vi "Default Instrument Setup.vi"(8 "error in (no error)":errorcluster, 11 "VISA resource name":refnum<visa-resource-name>) -> (0 "error out":errorcluster, 3 "VISA resource name out":refnum<visa-resource-name>)   [LabVIEW 2021, in "Siglent SDS 1000 2000 Series.lvlib"]
doc: "This Utility VI sends a default command string to the instrument whenever a new VISA session is opened, or the instrument is reset. This VI is intended to be used as a subVI for the <B>Initialize</B> and <B>Reset</B> VI's. Altering this VI could cause these two VI's to operate incorrectly."
uses:
  <instrlib>/Siglent SDS 1000 2000 Series/Siglent SDS 1000 2000 Series.lvlib
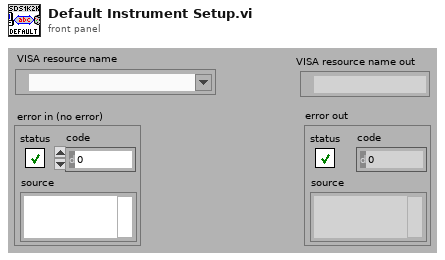
[diagram p1: front panel]
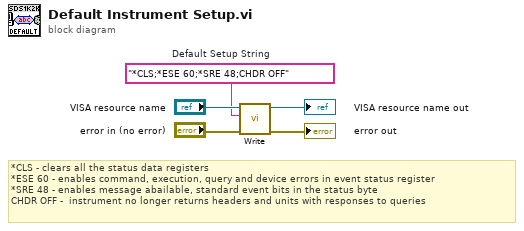
[diagram p0: block diagram]
diagram:
  w1 = "*CLS;*ESE 60;*SRE 48;CHDR OFF"  # Default Setup String
  # "*CLS - clears all the status data registers\n*ESE 60 - enables command, execution, query and device errors in event status register \n*SRE 48 - enables message abailable, standard event bits in the status byte\nCHDR OFF -  instrument no longer returns headers and units with responses to queries"
  n1 = call <instrlib>:"Write.vi"("error in (no error)"="error in (no error)", "Write Buffer"=w1, "VISA resource name"="VISA resource name") -> ("error out"=→"error out":errorcluster, "VISA resource name out"=→"VISA resource name out":refnum<visa-resource-name>)  [unwired: 6 in, 1 out]
